vi "WriteModeDM_DUAL.vi"(5 "Clear DM Voltage":bool, 6 "Flat File ON":bool, 9 "Amplitudes":dbl[](array[numeric]), 10 "Modes":i32[](array[numeric]), 11 "Device":i32) -> (0 "Voltage Map Out":dbl[](array[numeric]), 3 "Voltage Map":dbl[][](array[numeric]))   [LabVIEW 2014]
uses:
  <vilib>/Analysis/baseanly.llb/A x Vector.vi
  <vilib>/Analysis/NI_AALBase.lvlib
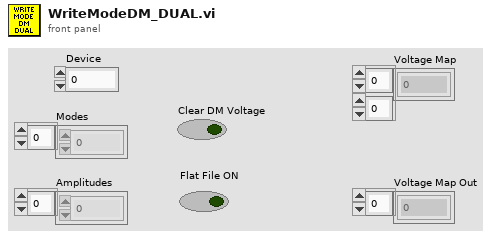
[diagram p1: front panel]
types:
  T1 = typedef "NI_Matrix.lvlib/RealMatrix.ctl" = dbl[][]
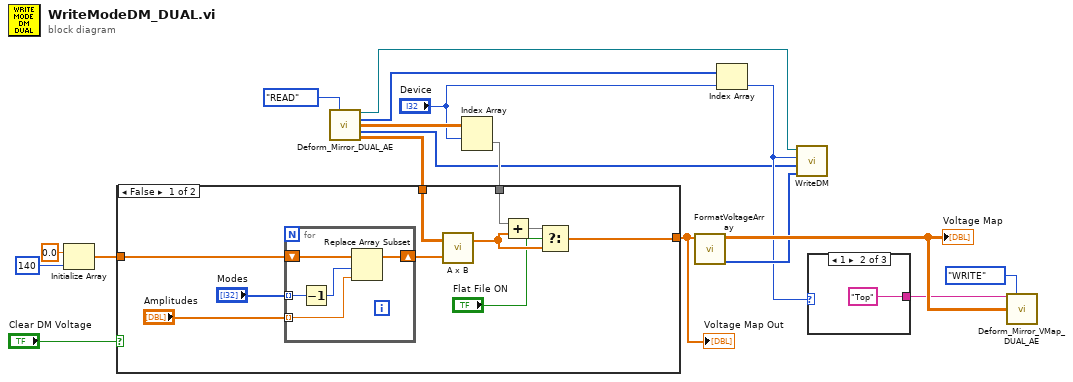
[diagram p0: block diagram]
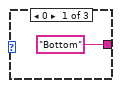
[diagram p3: hidden frame]
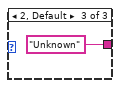
[diagram p4: hidden frame]
diagram:
  n1 = Initialize Array(0.0 ("element"), 140 ("dimension size")) -> (w13:dbl[])
  n2 = call "Deform_Mirror_DUAL_AE.vi"("Action"=enum16{"WRITE", "READ"}."READ" ("Enum")) -> ("Refnum Out"=w6:refnum<k7>, "IDs Out"=w7:i32[], "Flat Files Out"=w10:dbl[][], "Multi Map Data Out"=w3:i32[], "Mode Matrix Out"=w12:T1)  [unwired: 10 in]
  n3 = Index Array(array=w10, index (row)="Device") -> (element=w9:dbl[])  [unwired: 1 in]
  n4 = case shown="False" "Clear DM Voltage" {
    tunnel: w13 -> [w25 w34]
    tunnel: w12 -> [w24 _]
    tunnel: w9 -> [w20 _]
    tunnel: [w19 w34] -> w1
    frame False {
      n5 = for {
        tunnel: "Modes" -> [w32] mode=indexing
        tunnel: "Amplitudes" -> [w30] mode=indexing
        shift-right: [w29] -> w26
        shift-left: w25 -> [w33]
        n6 = Decrement(x=w32) -> (x-1=w31:i32)
        n7 = Replace Array Subset(array=w33, new element=w30, index=w31) -> (w29:dbl[])
      }
      n8 = call-poly <vilib>:"A x B.vi"("Vector"=w26, "A"=w24) -> ("A x Vector"=w22:dbl[])  [unwired: 1 out]
      n9 = Add(x=w20, y=w22) -> (x+y=w23:dbl[])
      n10 = Select(t=w23, s="Flat File ON", f=w22) -> (s? t:f=w19:dbl[])
    }
    frame True {
    }
  }
  "Voltage Map Out" <- w1
  n11 = call "FormatVoltageArray.vi"("Array in"=w1) -> ("Mirror Array"=w5:u16[], "Voltage Map"=w15:dbl[][])  [unwired: 9 in]
  "Voltage Map" <- w15
  n12 = Index Array(array=w7, index="Device") -> (element=w4:i32)
  n13 = call "WriteDM.vi"("reference in"=w6, "nDevId"=w4, "MultiDM  Mapping"=w3, "Voltage Array in"=w5) -> ()  [unwired: 2 in, 2 out]
  n14 = case shown="1" w4 {
    tunnel: ["Bottom" "Top" "Unknown"] -> w2
    frame 0 {
    }
    frame 1 {
    }
    frame 2, Default {
    }
  }
  n15 = call "Deform_Mirror_VMap_DUAL_AE.vi"("Mirror ID"=w2, "Enum"=enum16{"WRITE", "READ"}."WRITE", "V Map In"=w15) -> ()  [unwired: 12 in, 1 out]
